vi "initialize redirection.vi"(11 "Oauth2":refnum<class "Oauth2.lvclass">) -> (1 "error out":errorcluster, 3 "Redirect URI":string="http://localhost:58888/Oauth2/Redirect")   [LabVIEW 2017, in "Oauth2.lvclass"]
uses:
  Oauth2.lvclass
  <vilib>/LabVIEW Open Source Project/OpenURI/uri/URI.lvclass
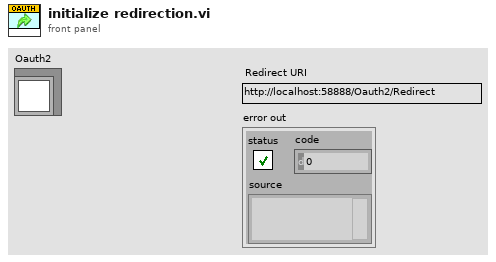
[diagram p1: front panel]
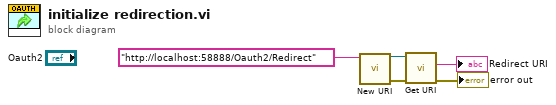
[diagram p0: block diagram]
diagram:
  n1 = call <vilib>:"New URI.vi"("URI"="http://localhost:58888/Oauth2/Redirect") -> ("error out"=w4:errorcluster, "URI"=w3:refnum<class "URI.lvclass">)  [unwired: 9 in]
  n2 = call <vilib>:"Get URI.vi"("error in (no error)"=w4, "URI in"=w3) -> ("error out"=→"error out":errorcluster, "URI String"=→"Redirect URI":string)  [unwired: 7 in, 1 out]
